vi "Publisher Do.vi"(8 "error in (no error)":errorcluster, 10 "Actor in":refnum<class "Publisher.lvclass">, 11 "Launch Subscriber Msg":refnum<class "Launch Subscriber Msg.lvclass">) -> (0 "error out":errorcluster, 2 "Actor out":refnum<class "Publisher.lvclass">)   [LabVIEW 2020, in "Publisher.lvlib" / "Launch Subscriber Msg.lvclass"]
doc: "This VI delivers the message to the actor by calling the appropriate method(s) on the actor."
uses:
  Launch Subscriber Msg.lvclass
  Publisher/Publisher.lvclass
  Launch Subscriber Msg.lvclass/Launch Subscriber Msg.ctl
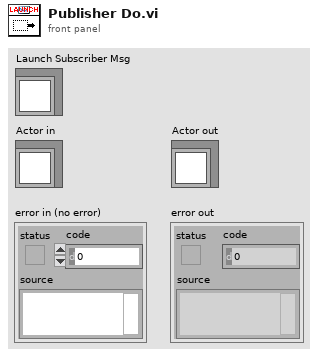
[diagram p1: front panel]
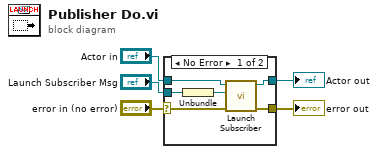
[diagram p0: block diagram]
diagram:
  n1 = case shown="No Error" "error in (no error)" {
    selector: "error in (no error)" -> [w9 w13]
    tunnel: [w11 w13] -> w4
    tunnel: [w10 w12] -> w3
    tunnel: "Actor in" -> [w6 w12]
    tunnel: "Launch Subscriber Msg" -> [w8 _]
    frame No Error {
      n2 = Unbundle(w8) -> (w7:refnum<class "Actor.lvclass">)
      n3 = call "Launch Subscriber.vi"("error in (no error)"=w9, "Actor to Launch"=w7, "Publisher in"=w6) -> ("error out"=w11:errorcluster, "Publisher out"=w10:refnum<class "Publisher.lvclass">)  [unwired: 7 in]
    }
    frame Error {
    }
  }
  "error out" <- w4
  "Actor out" <- w3
